vi "Save with Temperature.vi"() -> ()   [LabVIEW 2016]
uses:
  <vilib>/Utility/file.llb/Write Delimited Spreadsheet (DBL).vi
  source/INST DRIVERS/DilutionFridge/MyTriton.lvlib
panel:
  out "Read Temperature":dbl
  in  "Save to buffer?":bool
  in  "Save now?":bool
  in  "file path (dialog if empty)":path
  out "Buffer size":i32
  out "output array":dbl[](array[numeric])
  in  "Manual T (K)":dbl
  in  "Manual Entry of Temperature?":bool
  out "error out":errorcluster
  in  "Boolean":bool
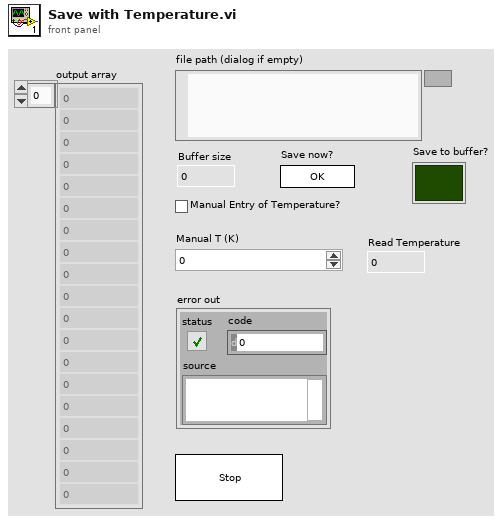
[diagram p1: front panel]
types:
  T1 = enum16{"Read", "Write", "ReadWrite", "BufferedRead", "BufferedReadWrite"}
  T2 = enum8{"Enabled", "Disabled", "Disabled and Grayed Out"}
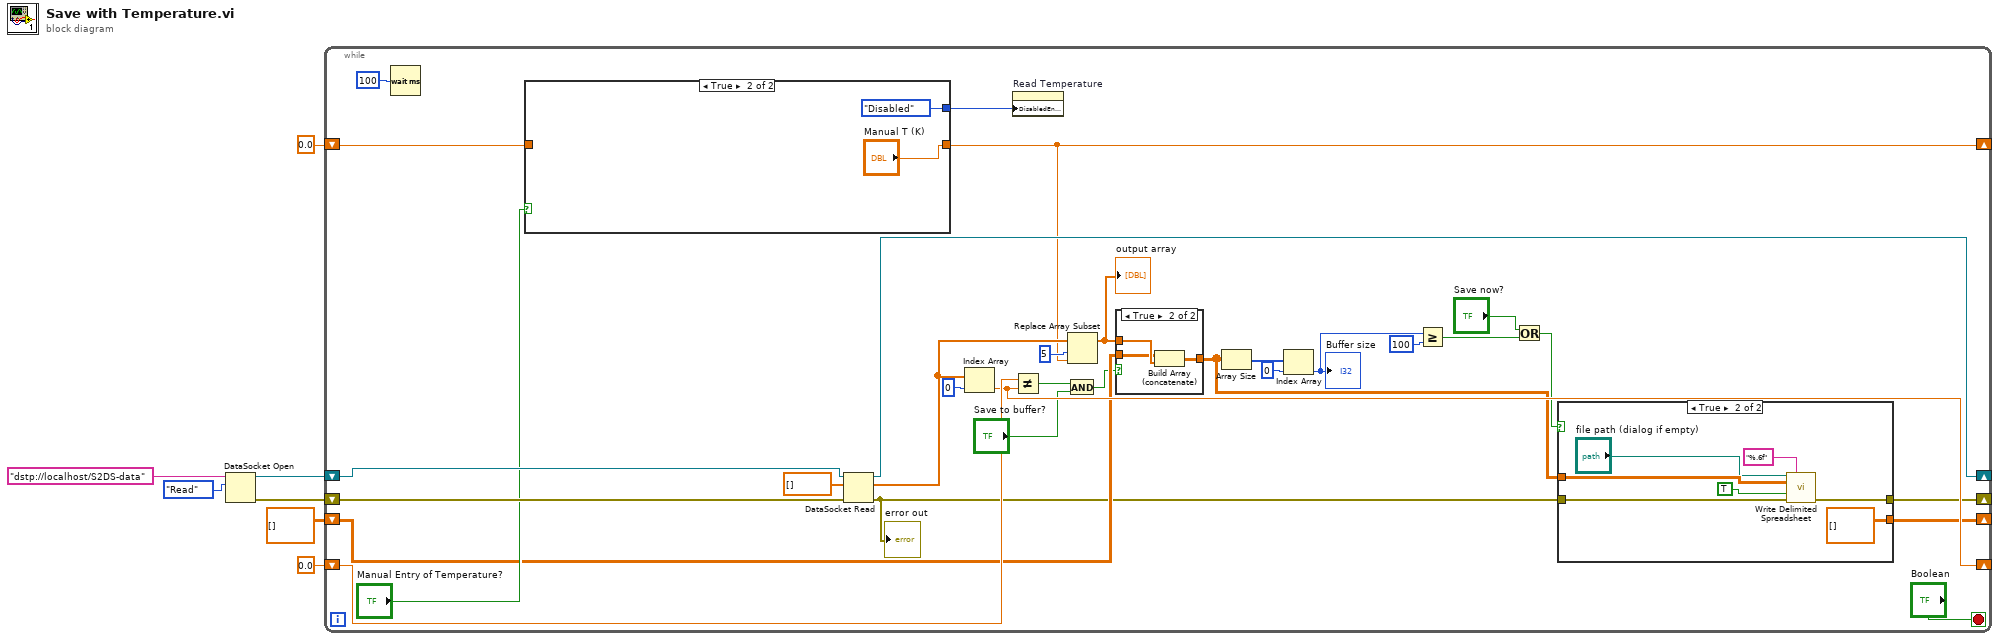
[diagram p0: block diagram]
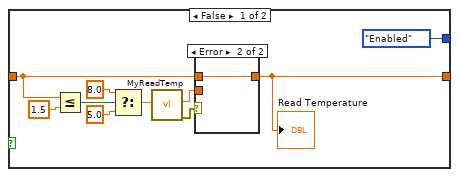
[diagram p4: hidden frame]
diagram:
  n1 = DataSocket Open(10:T1."Read" ("mode"), 11:"dstp://localhost/S2DS-data" ("URL")) -> (0:w4:errorcluster, 3:w5:refnum<k13>)  [unwired: 2 in]
  n2 = while {
    shift-right: [w35] -> _
    shift-left: w5 -> [w37]
    shift-right: [w15] -> _
    shift-left: w4 -> [w38]
    shift-right: [w30] -> _
    shift-left: 0.0 -> [w31]
    shift-right: [w25] -> _
    shift-left: 0.0 -> [w28]
    shift-right: [w18] -> _
    shift-left: dbl[][] [] -> [w23]
    stop <- "Boolean" stop-if-true
    n3 = Wait (ms)(milliseconds to wait=u32 100) -> ()  [unwired: 1 out]
    n4 = case shown="True" "Manual Entry of Temperature?" {
      tunnel: [w59 "Manual T (K)"] -> w25
      tunnel: w28 -> [w58 _]
      tunnel: [T2."Enabled" ("Disabled") T2."Disabled" ("Disabled")] -> w8
      frame False {
        n5 = Less Or Equal?(x=w58, y=1.5) -> (x <= y?=w56:bool)
        n6 = Select(t=8.0, s=w56, f=5.0) -> (s? t:f=w53:dbl)
        n7 = call "MyReadTemp.vi"("Temperature Channel"=w53) -> ("error out"=w61:errorcluster, "Temperature"=w60:dbl)  [unwired: 8 in, 1 out]
        n8 = case shown="Error" w61 {
          tunnel: [w62 w63] -> w59
          tunnel: w60 -> [w62 _]
          tunnel: w58 -> [_ w63]
          frame No Error {
          }
          frame Error {
          }
        }
        "Read Temperature" <- w59
      }
      frame True {
      }
    }
    n9 = DataSocket Read(8:w38, 10:dbl[] [], 11:w37) -> (0:w16:errorcluster, 2:w27:dbl[], 3:w35:refnum<k13>)  [unwired: 2 in, 4 out]
    "error out" <- w16
    n10 = Index Array(array=w27, index=0) -> (element=w30:dbl)
    n11 = property on="Read Temperature" class="DigNum (strict)"("DisabledEnum"=w8) -> ()  [unwired: 2 in, 2 out]
    n12 = Not Equal?(x=w31, y=w30) -> (x != y?=w11:bool)
    n13 = And(x=w11, y="Save to buffer?") -> (x .and. y?=w9:bool)
    n14 = Replace Array Subset(array=w27, new element=w25, index=5) -> (w24:dbl[])
    "output array" <- w24
    n15 = case shown="True" w9 {
      tunnel: w24 -> [_ w51]
      tunnel: w23 -> [w48 w50]
      tunnel: [w48 w49] -> w17
      frame False {
      }
      frame True {
        n16 = Build Array (concatenate)(w50, w51) -> (w49:dbl[][])
      }
    }
    n17 = Array Size(array=w17) -> (size(s)=w22:i32[])
    n18 = Index Array(array=w22, index=0) -> (element=w20:i32)
    "Buffer size" <- w20
    n19 = Greater Or Equal?(x=w20, y=100) -> (x >= y?=w13:bool)
    n20 = Or(x="Save now?", y=w13) -> (x .or. y?=w12:bool)
    n21 = case shown="True" w12 {
      tunnel: [w40 dbl[][] []] -> w18
      tunnel: w17 -> [w40 w46]
      tunnel: w16 -> [w39 w45]
      tunnel: [w39 w44] -> w15
      frame False {
      }
      frame True {
        n22 = call-poly <vilib>:"Write Delimited Spreadsheet.vi"("file path (dialog if empty)"="file path (dialog if empty)", "format (%.3f)"="%.6f", "2D data"=w46, "append to file? (new file:F)"=TRUE, "error in (no error)"=w45) -> ("error out"=w44:errorcluster)  [unwired: 9 in, 1 out]
      }
    }
  }
